vi "Sweep_Process.vi"(8 "错误输入（无错误）":errorcluster, 9 "MPM":refnum<k24>[](array[refnum]), 10 "TSL":refnum<k24>, 11 "SPU":refnum<k24>) -> (0 "error out":errorcluster, 1 "MPM out":refnum<k24>[](array[refnum]), 2 "TSL out":refnum<k24>, 3 "SPU out":refnum<k24>)   [LabVIEW 2017]
doc: "Sweep"
uses:
  D:/test/ILSTS/LV_IL_Sample/DLL/InstrumentDLL.dll
  DLL/InstrumentDLL.dll
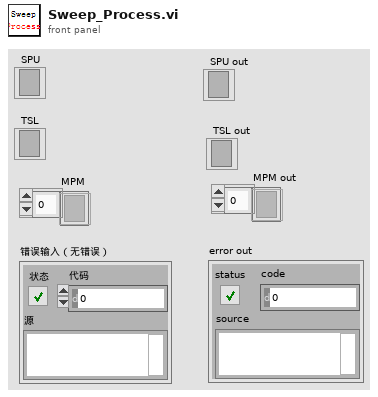
[diagram p1: front panel]
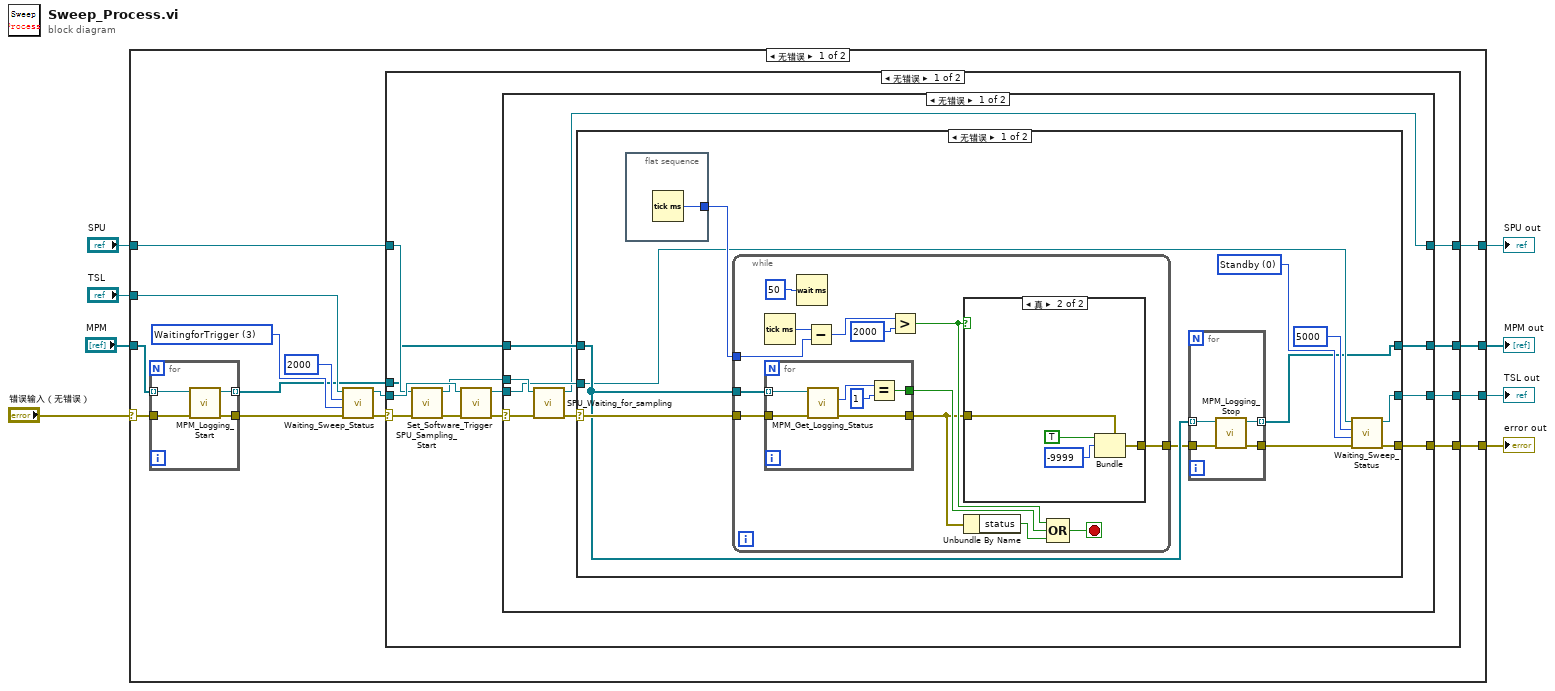
[diagram p0: block diagram]
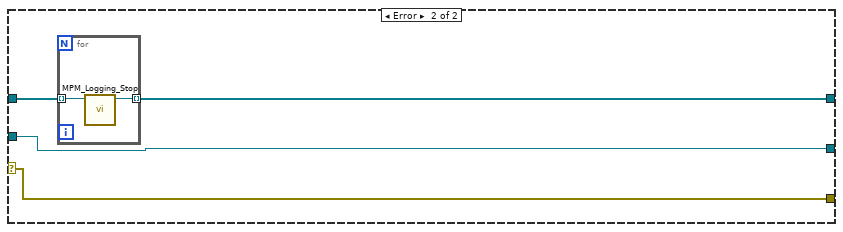
[diagram p3: hidden frame]
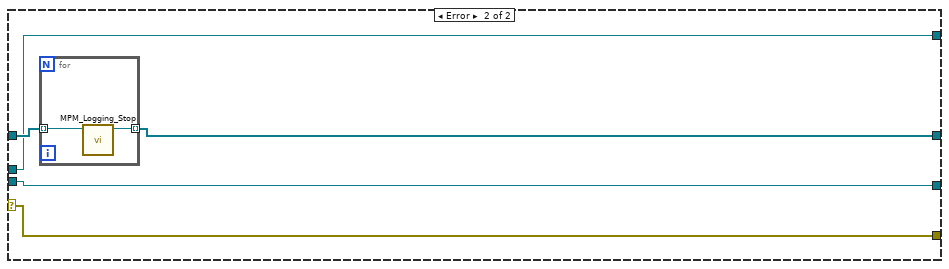
[diagram p4: hidden frame]
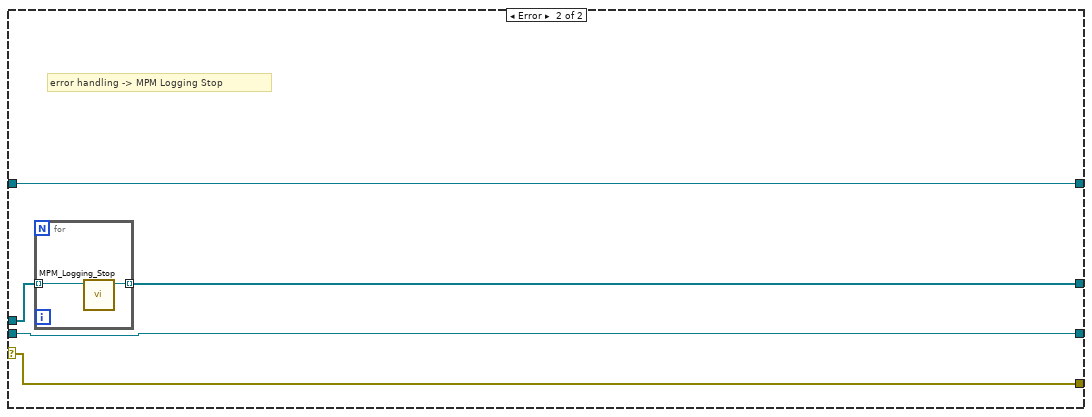
[diagram p5: hidden frame]
diagram:
  n1 = case shown="无错误" "错误输入（无错误）" {
    selector: "错误输入（无错误）" -> [w13 w111]
    tunnel: "SPU" -> [w22 w110]
    tunnel: "TSL" -> [w16 w109]
    tunnel: [w15 w111] -> w6
    tunnel: "MPM" -> [w14 w108]
    tunnel: [w12 w110] -> w3
    tunnel: [w11 w109] -> w2
    tunnel: [w9 w108] -> w1
    frame No Error {
      w19 = 3 items=["Standby", "Running", "Pausing", "WaitingforTrigger", "Returning"] ("status")
      n2 = for {
        tunnel: w14 -> [w107] mode=indexing
        tunnel: w13 -> [w106]
        tunnel: [w105] -> w17
        tunnel: [w104] -> w10 mode=indexing
        n3 = call "MPM_Logging_Start.vi"("error in (no error)"=w106, ".NET Reference in"=w107) -> ("error out"=w105:errorcluster, "Reference out"=w104:refnum<k24>)  [unwired: 8 in]
      }
      n4 = call "Waiting_Sweep_Status.vi"("error in (no error)"=w17, "status"=w19, "Wait time(msec)"=2000, ".NET Reference in"=w16) -> ("error out"=w20:errorcluster, "Reference out"=w21:refnum<k24>)  [unwired: 6 in]
      n5 = case shown="无错误" w20 {
        selector: w20 -> [w32 w100]
        tunnel: w21 -> [w33 w97]
        tunnel: w22 -> [w31 w99]
        tunnel: w10 -> [w30 w101]
        tunnel: [w26 w100] -> w15
        tunnel: [w25 w99] -> w12
        tunnel: [w24 w97] -> w11
        tunnel: [w23 w98] -> w9
        frame No Error {
          n6 = call "SPU_Sampling_Start.vi"("错误输入（无错误）"=w32, "引用"=w31) -> ("error IO"=w34:errorcluster, "引用输出"=w28:refnum<k24>)  [unwired: 7 in]
          n7 = call "Set_Software_Trigger.vi"("error in (no error)"=w34, ".NET Reference in"=w33) -> ("error out"=w29:errorcluster, "Reference out"=w27:refnum<k24>)  [unwired: 8 in]
          n8 = case shown="无错误" w29 {
            selector: w29 -> [w43 w93]
            tunnel: w30 -> [w40 w94]
            tunnel: w28 -> [w42 w92]
            tunnel: w27 -> [w39 w90]
            tunnel: [w38 w93] -> w26
            tunnel: [w37 w92] -> w25
            tunnel: [w36 w90] -> w24
            tunnel: [w35 w91] -> w23
            frame No Error {
              n9 = call "SPU_Waiting_for_sampling.vi"("错误输入（无错误）"=w43, "引用"=w42) -> ("error IO"=w41:errorcluster, "引用输出"=w37:refnum<k24>)  [unwired: 7 in]
              n10 = case shown="无错误" w41 {
                selector: w41 -> [w54 w86]
                tunnel: w40 -> [w52 w87]
                tunnel: w39 -> [w48 w84]
                tunnel: [w47 w86] -> w38
                tunnel: [w45 w84] -> w36
                tunnel: [w44 w85] -> w35
                frame No Error {
                  w50 = 0 items=["Standby", "Running", "Pausing", "WaitingforTrigger", "Returning"] ("status")
                  n11 = flat-sequence {
                    tunnel: [w59] -> w53
                    frame #0 {
                      n12 = Tick Count (ms)() -> (millisecond timer value=w59:u32)
                    }
                  }
                  n13 = while {
                    tunnel: w52 -> [w72]
                    tunnel: w54 -> [w71]
                    tunnel: w53 -> [w68]
                    tunnel: [w60] -> w46
                    stop <- w64 stop-if-true
                    n14 = Tick Count (ms)() -> (millisecond timer value=w69:u32)
                    n15 = for {
                      tunnel: w72 -> [w83] mode=indexing
                      tunnel: w71 -> [w82]
                      tunnel: [w79] -> w65
                      tunnel: [w78] -> w61
                      n16 = call "MPM_Get_Logging_Status.vi"("error in (no error)"=w82, ".NET Reference in"=w83) -> ("error out"=w78:errorcluster, "status out"=w81:i32)  [unwired: 6 in, 2 out]
                      n17 = Equal?(x=w81, y=1) -> (x = y?=w79:bool)
                    }
                    n18 = Wait (ms)(milliseconds to wait=u32 50 ("等待时间（毫秒）")) -> ()  [unwired: 1 out]
                    n19 = Subtract(x=w69, y=w68) -> (x-y=w67:u32)
                    n20 = Greater?(x=w67, y=u32 2000) -> (0:w62:bool)
                    n21 = case shown="真" w62 {
                      tunnel: w61 -> [w73 w77]
                      tunnel: [w73 w74] -> w60
                      frame False {
                      }
                      frame True {
                        n22 = Bundle(cluster=w77, "status"=TRUE, "code"=-9999) -> (w74:errorcluster)  [unwired: 1 in]
                      }
                    }
                    n23 = Unbundle By Name(w61) -> ("status"=w63:bool)
                    n24 = Compound Arithmetic op=OR ("复合运算")(w62, w65, w63) -> (w64:bool)
                  }
                  n25 = for {
                    tunnel: w52 -> [w58] mode=indexing
                    tunnel: [w57] -> w51
                    tunnel: w46 -> [w56]
                    tunnel: [w55] -> w44 mode=indexing
                    n26 = call "MPM_Logging_Stop.vi"("error in (no error)"=w56, ".NET Reference in"=w58) -> ("error out"=w57:errorcluster, "Reference out"=w55:refnum<k24>)  [unwired: 8 in]
                  }
                  n27 = call "Waiting_Sweep_Status.vi"("error in (no error)"=w51, "status"=w50, "Wait time(msec)"=5000, ".NET Reference in"=w48) -> ("error out"=w47:errorcluster, "Reference out"=w45:refnum<k24>)  [unwired: 6 in]
                }
                frame Error {
                  n28 = for {
                    tunnel: w87 -> [w89] mode=indexing
                    tunnel: [w88] -> w85 mode=indexing
                    n29 = call "MPM_Logging_Stop.vi"(".NET Reference in"=w89) -> ("Reference out"=w88:refnum<k24>)  [unwired: 9 in, 1 out]
                  }
                }
              }
            }
            frame Error {
              n30 = for {
                tunnel: w94 -> [w96] mode=indexing
                tunnel: [w95] -> w91 mode=indexing
                n31 = call "MPM_Logging_Stop.vi"(".NET Reference in"=w96) -> ("Reference out"=w95:refnum<k24>)  [unwired: 9 in, 1 out]
              }
            }
          }
        }
        frame Error {
          # "error handling -> MPM Logging Stop"
          n32 = for {
            tunnel: w101 -> [w103] mode=indexing
            tunnel: [w102] -> w98 mode=indexing
            n33 = call "MPM_Logging_Stop.vi"(".NET Reference in"=w103) -> ("Reference out"=w102:refnum<k24>)  [unwired: 9 in, 1 out]
          }
        }
      }
    }
    frame Error {
    }
  }
  "error out" <- w6
  "SPU out" <- w3
  "TSL out" <- w2
  "MPM out" <- w1
